vi "输入数据解析.vi"(0 "单个参数补充":dbl, 1 "从板号":dbl=1.0, 2 "主板二维码":string="BNET01", 3 "从板二维码":string="BNET01", 5 "主板引用":refnum<vi>, 7 "从板引用":refnum<vi>, 9 "主板选项":string="三级故障阀值", 11 "枚举":enum16{"主板", "从板"}(ring), 12 "快换":bool caption="快换写入") -> (4 "输出数组":dbl[][](array[numeric]), 6 "数组长度":dbl[](array[numeric]), 8 "循环次数":i32, 10 "命令":u32, 14 "名称":string[](array[string]), 15 "命令序号":u32[](array[numeric]))   [LabVIEW 2013]
panel:
  out "从板信息":T1
  out "主板数据":T2
  out "低位子数组 18":i32[](array[numeric])
  out "低位子数组 17":i32[](array[numeric])
  out "低位子数组 16":i32[](array[numeric])
  out "低位子数组 15":i32[](array[numeric])
  out "低位子数组 14":i32[](array[numeric])
  out "低位子数组 13":i32[](array[numeric])
  out "低位子数组 12":i32[](array[numeric])
  out "低位子数组 11":i32[](array[numeric])
  out "低位子数组 10":i32[](array[numeric])
  out "低位子数组 9":i32[](array[numeric])
  out "低位子数组 8":i32[](array[numeric])
  out "低位子数组 7":i32[](array[numeric])
  out "低位子数组 6":i32[](array[numeric])
  out "低位子数组 5":i32[](array[numeric])
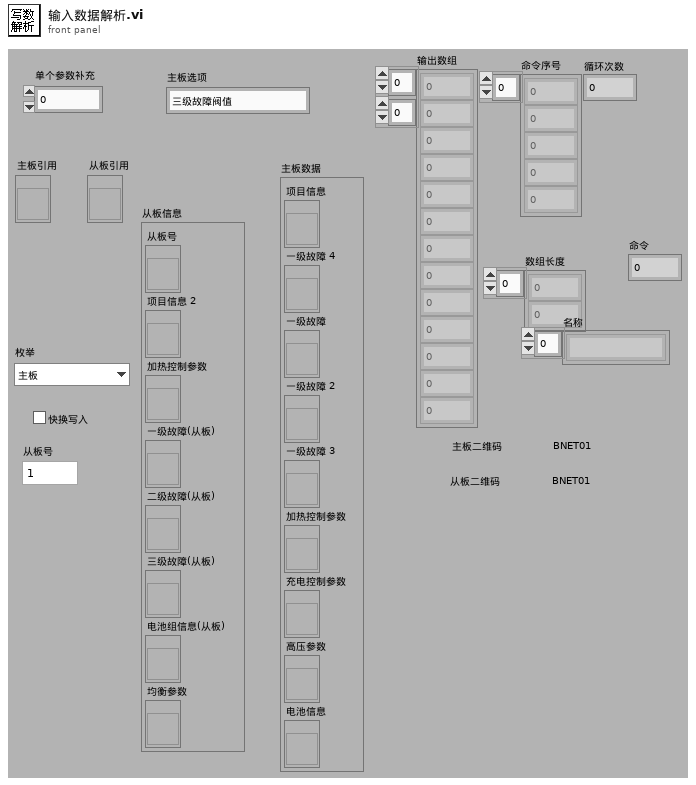
[diagram p1: front panel]
types:
  T1 = cluster{"从板号":refnum<vi>, "项目信息 2":refnum<vi>, "加热控制参数":refnum<vi>, "一级故障(从板)":refnum<vi>, "二级故障(从板)":refnum<vi>, "三级故障(从板)":refnum<vi>, "电池组信息(从板)":refnum<vi>, "均衡参数":refnum<vi>}
  T2 = cluster{"项目信息":refnum<vi>, "一级故障 4":refnum<vi>, "一级故障":refnum<vi>, "一级故障 2":refnum<vi>, "一级故障 3":refnum<vi>, "加热控制参数":refnum<vi>, "充电控制参数":refnum<vi>, "高压参数":refnum<vi>, "电池信息":refnum<vi>}
  T3 = cluster{"电池额定容量(A)":dbl, "使用者":dbl, "电池实际容量(A)":dbl, "车架(牌)号":string, "配置文件版本":string, "SOH(%)":dbl, "SOC(%)":dbl, "产品编号":string, "系统时钟":string}
  T4 = cluster{"总电压过高":dbl, "整组电压不均衡":dbl, "SOC过高":dbl, "单体电压过高":dbl, "总电压过低":dbl, "温度过高":dbl, "温度过低":dbl, "单组电压不均衡":dbl, "整组温度不均衡":dbl, "单组温度不均衡":dbl, "单体电压过低":dbl, "充电电流过高":dbl, "放电电流过高":dbl, "SOC过低":dbl, "内阻过大":dbl, "极柱温度过高":dbl, "SOH过低":dbl}
  T5 = cluster{"风机开启温度":dbl, "风机关闭温度":dbl, "加热开启温度":dbl, "加热关闭温度":dbl, "风机开启温差":dbl, "风机关闭温差":dbl, "加热关闭温差":dbl}
  T6 = cluster{"最大允许单体电压":dbl, "最大允许总电压":dbl, "最小允许单体电压":dbl, "最大允许充电电流":dbl, "最小允许充电电流":dbl, "最大允许充电温度":dbl, "最小允许充电温度":dbl, "电流步长":dbl}
  T7 = cluster{"电池串联":dbl, "电池并联":dbl, "累计放电总安时":dbl, "电池包额定容量":dbl, "电池包额定能量":dbl, "电池包额定总电压":dbl, "累计充电总安时":dbl, "电池充满次数":dbl, "电池放空次数":dbl, "电池充电次数":dbl, "电池生产日期":string, "电池厂家":string, "电池类型":string, "电池包组号":string, "电池包产权标识":string, "电池应用车型":string, "实际容量":dbl}
  T8 = cluster{"电压过高":dbl, "电压过低":dbl, "温度过高":dbl, "温度过低":dbl, "电压不均衡(V)":dbl, "温度不均衡":dbl, "SOC过低":dbl}
  T9 = cluster{"串联数":dbl, "并联数":dbl, "电池厂家":dbl, "电池类型":dbl, "额定能量":dbl, "额定容量":dbl, "实际容量":dbl, "额定总压":dbl, "产权标识":dbl, "应用车型":dbl, "电池包组号":dbl, "SOC":dbl, "充电总安时":dbl, "放电总这时":dbl, "放空次数":dbl, "充满次数":dbl, "充电次数":dbl, "车牌号":string, "生产日期":string, "最大允许单体电压":dbl, "最大允许总电压":dbl, "最大允许温度":dbl, "最小允许温度":dbl, "最大允许充电电流":dbl, "最小允许充电电流":dbl, "最小允许单体电压":dbl, "电流步长":dbl, "电池包序号":dbl}
  T10 = cluster{"充电结束电压(90%)":sgl, "充电结束电压(91%)":sgl, "充电结束电压(92%)":sgl, "充电结束电压(93%)":sgl, "充电结束电压(94%)":sgl, "均衡计算-电压高阀值1级":sgl, "均衡计算-电压高阀值2级":sgl, "均衡计算-电压低阀值1级":sgl, "均衡计算-电压低阀值2级":sgl, "均衡计算-最低电压阀值":sgl, "均衡停止-最低电压阀值":sgl, "均衡计算-电压极差阀值":sgl, "充电结束电压(95%)":sgl, "充电结束电压(96%)":sgl, "充电结束电压(97%)":sgl, "充电结束电压(98%)":sgl, "充电结束电压(99%)":sgl, "充电结束电压(100%)":sgl}
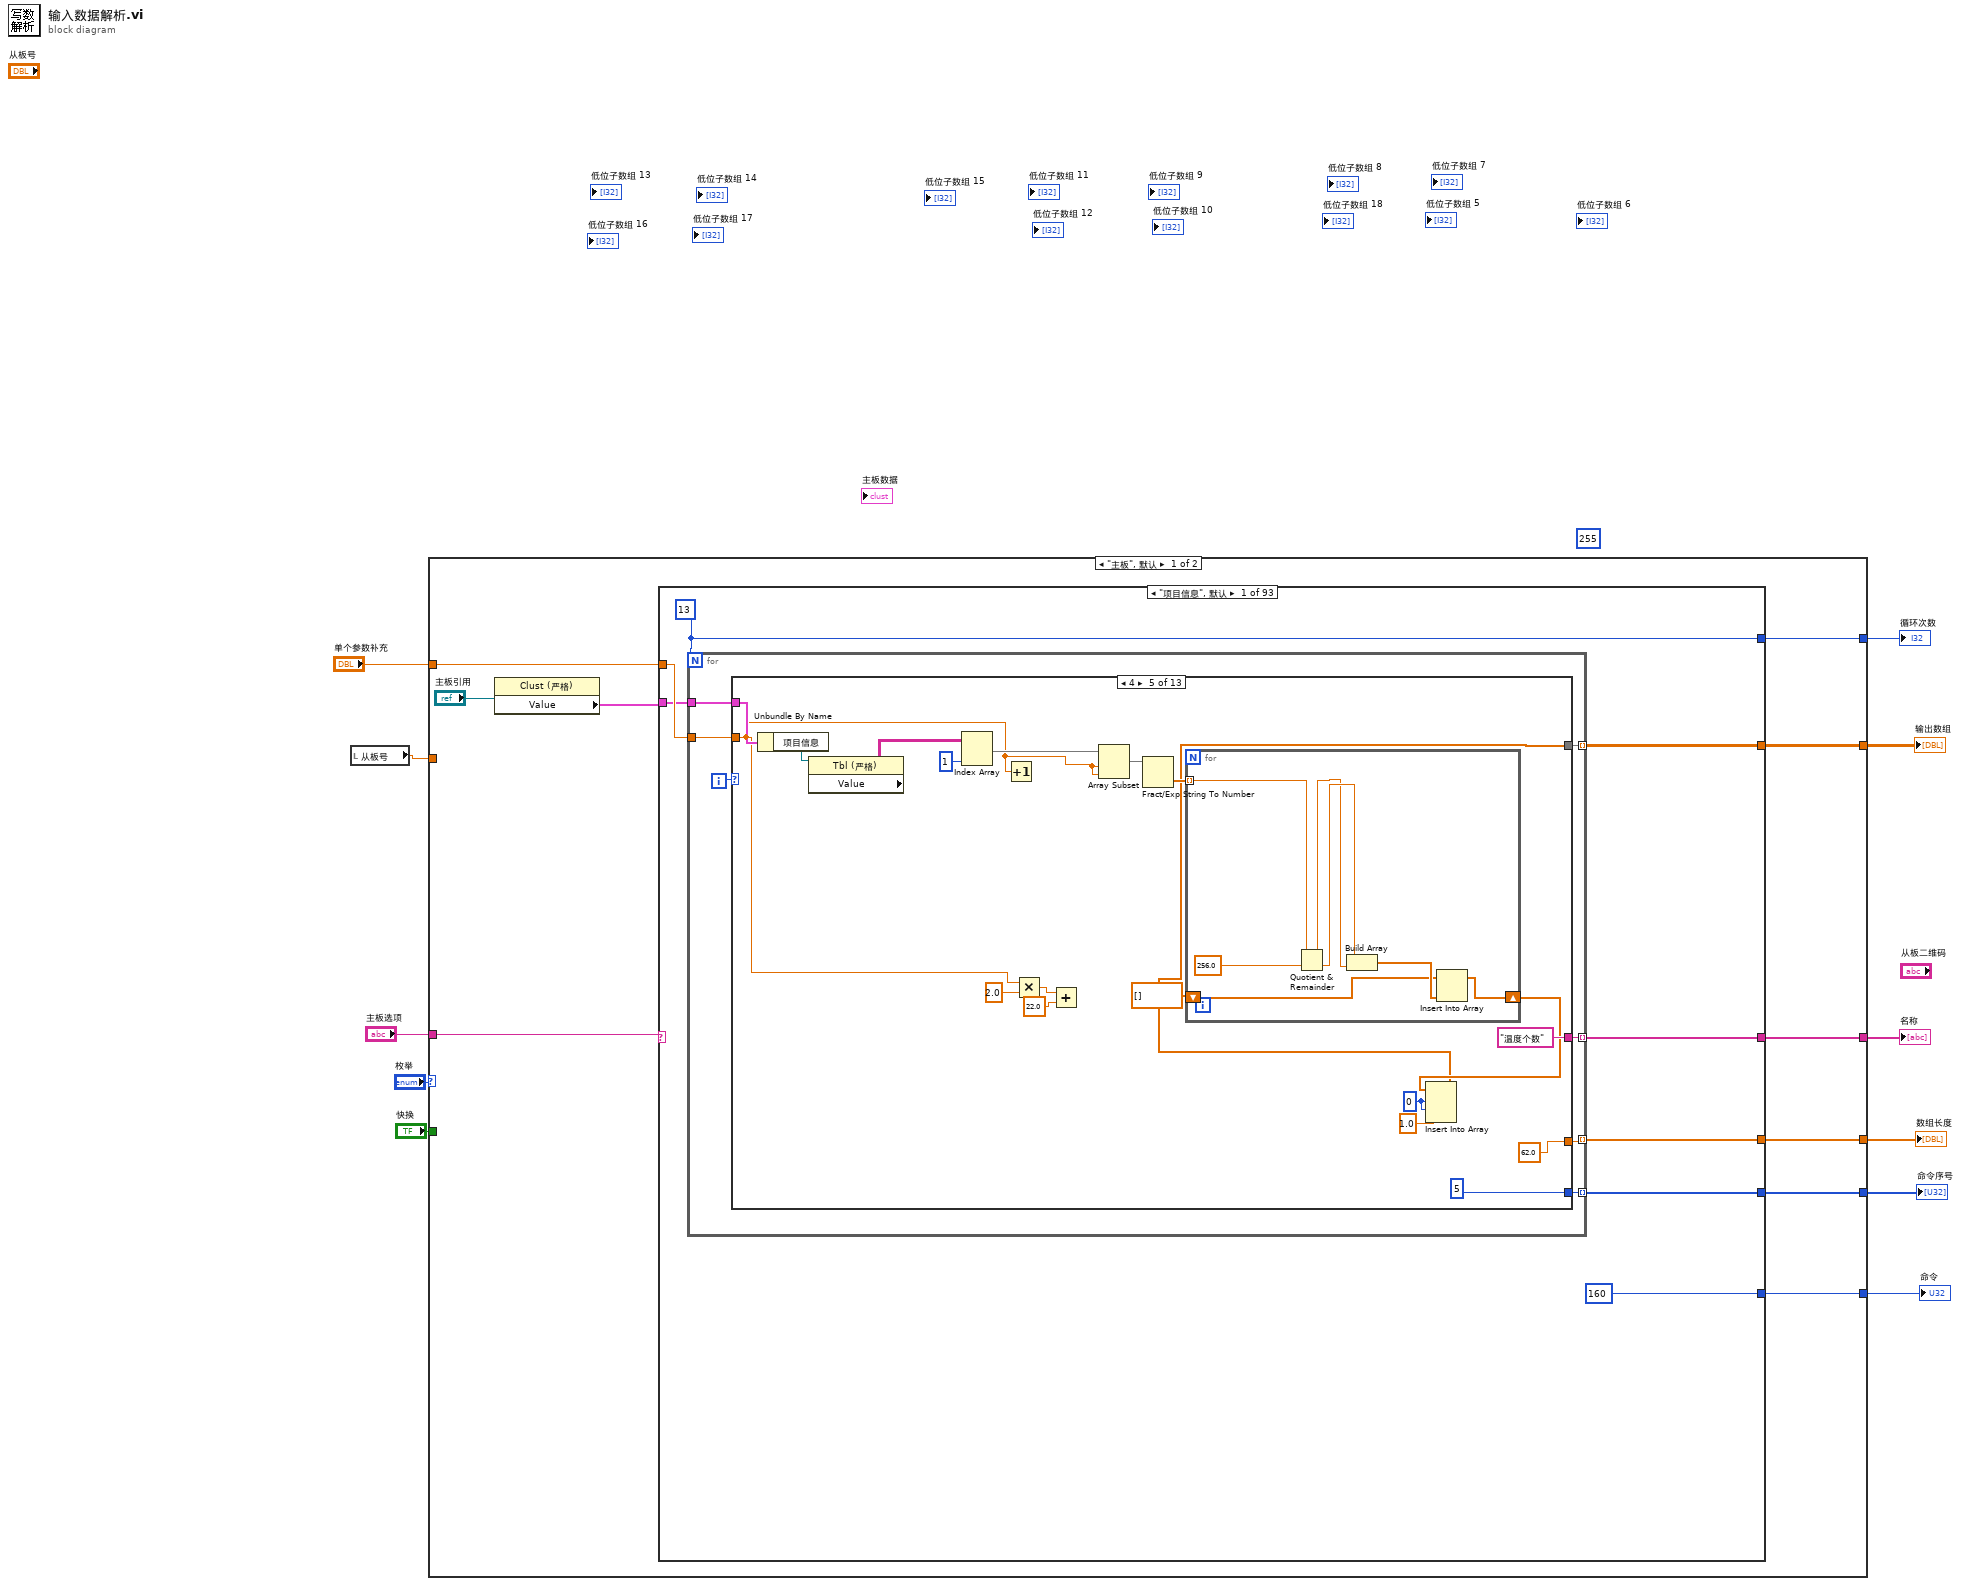
[diagram p0: block diagram]
diagram:
  (unwired) 255 ("高字节1")
  n1 = local read "从板号"() -> (w3:dbl)
  n2 = case shown="\"主板\", 默认" "枚举" {
    tunnel: "主板选项" -> [w21 w14872]
    tunnel: "单个参数补充" -> [w20 w14867]
    tunnel: [w19 w14871] -> w9
    tunnel: [w18 w14869] -> w8
    tunnel: [w17 w14868] -> w7
    tunnel: [w16 w14870] -> w6
    tunnel: "快换" -> [_ w14866]
    tunnel: w3 -> [_ w14865]
    tunnel: [w13 w14862] -> w2
    tunnel: [w12 w14861] -> w1
    frame "主板", Default {
      n3 = property class="Clust (严格)"(reference="主板引用") -> ("Value"=w14:T2)  [unwired: 1 in, 2 out]
      n4 = case shown="\"项目信息\", 默认" w21 {
        tunnel: w20 -> [w29 w289 _ _ w567 w599 w630 w651 w689 _ _ _ _ _ _ _ _ _ _ _ _ _ _ _ _ _ _ _ _ _ _ _ _ _ _ _ _ _ _ _ _ _ _ _ _ _ _ _ _ _ _ _ _ _ _ _ _ _ _ _ _ _ _ _ _ _ _ _ _ _ _ _ _ _ _ _ _ _ _ _ _ _ _ _ _ _ _ _ _ _ _ _ _]
        tunnel: w14 -> [w27 w287 w548 _ w586 w616 w643 w671 w702 w730 w767 w782 w806 _ w838 w856 w863 w1006 w1237 w1468 w1699 w1930 w2161 w2392 w2623 w2854 w3085 w3316 w3547 w3778 w4008 w4238 w4468 w4699 w4930 w5161 w5390 w5619 w5848 w6078 w6308 w6538 w6767 w6996 w7225 w7455 w7685 w7915 w8145 w8375 w8605 w8834 w9063 w9292 w9522 w9752 w9982 w10212 w10442 w10672 w10891 w11109 w11329 w11544 w11759 w11970 w12184 w12398 w12612 w12755 w12914 w12936 w12958 w12980 w13002 w13024 w13046 w13068 w13077 w13152 w13257 w13362 w13467 w13572 w13677 w13782 w13887 w13992 w14144 w14301 w14438 w14575 w14710]
        tunnel: [w28 w288 w535 w554 w571 w609 w636 w657 w683 w718 w738 w773 w789 w813 w829 w844 w867 w1010 w1241 w1472 w1703 w1934 w2165 w2396 w2627 w2858 w3089 w3320 w3551 w3782 w4012 w4242 w4472 w4703 w4934 w5165 w5394 w5623 w5852 w6082 w6312 w6542 w6771 w7000 w7229 w7459 w7689 w7919 w8149 w8379 w8609 w8838 w9067 w9296 w9526 w9756 w9986 w10216 w10446 w10676 w10895 w11113 w11333 w11548 w11763 w11974 w12188 w12402 w12616 w12759 w12918 w12940 w12962 w12984 w13006 w13028 w13050 w13072 w13084 w13159 w13264 w13369 w13474 w13579 w13684 w13789 w13894 w13994 w14146 w14303 w14440 w14577 w14709] -> w19
        tunnel: [w26 w286 w536 w555 w576 w606 w633 w662 w693 w716 w736 w771 w787 w811 w827 w842 u32[] [1] u32[] [1] u32[] [1] u32[] [1] u32[] [2] u32[] [3] u32[] [2] u32[] [3] u32[] [2] u32[] [3] u32[] [1] u32[] [2] u32[] [3] u32[] [1] u32[] [2] u32[] [3] u32[] [1] u32[] [2] u32[] [3] u32[] [1] u32[] [2] u32[] [3] u32[] [1] u32[] [2] u32[] [3] u32[] [1] u32[] [2] u32[] [3] u32[] [1] u32[] [2] u32[] [3] u32[] [1] u32[] [2] u32[] [3] u32[] [1] u32[] [2] u32[] [3] u32[] [1] u32[] [2] u32[] [3] u32[] [1] u32[] [2] u32[] [3] u32[] [1] u32[] [2] u32[] [3] u32[] [1] u32[] [2] u32[] [3] u32[] [1] u32[] [2] u32[] [3] u32[] [2] u32[] [3] u32[] [1] u32[] [1] u32[] [1] u32[] [1] u32[] [1] u32[] [1] u32[] [1] u32[] [1] u32[] [2] u32[] [2] u32[] [2] u32[] [2] u32[] [2] u32[] [2] u32[] [2] u32[] [2] u32[] [2] w13996 w14148 w14305 w14442 w14579 w14711] -> w18
        tunnel: [w25 w285 w537 w556 w578 w608 w635 w664 w695 w717 w737 w772 w788 w812 w828 w843 dbl[] [28.0] dbl[] [28.0] dbl[] [28.0] dbl[] [28.0] dbl[] [28.0] dbl[] [28.0] dbl[] [28.0] dbl[] [28.0] dbl[] [28.0] dbl[] [28.0] dbl[] [28.0] dbl[] [28.0] dbl[] [28.0] dbl[] [28.0] dbl[] [28.0] dbl[] [28.0] dbl[] [28.0] dbl[] [28.0] dbl[] [28.0] dbl[] [28.0] dbl[] [28.0] dbl[] [28.0] dbl[] [28.0] dbl[] [28.0] dbl[] [28.0] dbl[] [28.0] dbl[] [28.0] dbl[] [28.0] dbl[] [28.0] dbl[] [28.0] dbl[] [28.0] dbl[] [28.0] dbl[] [28.0] dbl[] [28.0] dbl[] [28.0] dbl[] [28.0] dbl[] [28.0] dbl[] [28.0] dbl[] [28.0] dbl[] [28.0] dbl[] [28.0] dbl[] [28.0] dbl[] [28.0] dbl[] [28.0] dbl[] [28.0] dbl[] [28.0] dbl[] [28.0] dbl[] [28.0] dbl[] [28.0] dbl[] [28.0] dbl[] [28.0] dbl[] [28.0] dbl[] [28.0] dbl[] [28.0] dbl[] [7.0] dbl[] [7.0] dbl[] [7.0] dbl[] [7.0] dbl[] [7.0] dbl[] [7.0] dbl[] [7.0] dbl[] [7.0] dbl[] [14.0] dbl[] [14.0] dbl[] [14.0] dbl[] [14.0] dbl[] [14.0] dbl[] [14.0] dbl[] [14.0] dbl[] [14.0] dbl[] [14.0] w13997 w14149 w14306 w14443 w14580 w14712] -> w17
        tunnel: [u32 160 ("命令序号") u32 160 ("命令序号") u32 160 ("命令序号") u32 172 ("命令序号") u32 160 ("命令序号") u32 160 ("命令序号") u32 160 ("命令序号") u32 160 ("命令序号") u32 160 ("命令序号") u32 160 ("命令序号") u32 160 ("命令序号") u32 160 ("命令序号") u32 160 ("命令序号") u32 160 ("命令序号") u32 160 ("命令序号") u32 160 ("命令序号") u32 161 ("命令序号") u32 161 ("命令序号") u32 161 ("命令序号") u32 161 ("命令序号") u32 161 ("命令序号") u32 161 ("命令序号") u32 161 ("命令序号") u32 161 ("命令序号") u32 161 ("命令序号") u32 161 ("命令序号") u32 161 ("命令序号") u32 161 ("命令序号") u32 161 ("命令序号") u32 161 ("命令序号") u32 161 ("命令序号") u32 161 ("命令序号") u32 161 ("命令序号") u32 161 ("命令序号") u32 161 ("命令序号") u32 161 ("命令序号") u32 161 ("命令序号") u32 161 ("命令序号") u32 161 ("命令序号") u32 161 ("命令序号") u32 161 ("命令序号") u32 161 ("命令序号") u32 161 ("命令序号") u32 161 ("命令序号") u32 161 ("命令序号") u32 161 ("命令序号") u32 161 ("命令序号") u32 161 ("命令序号") u32 161 ("命令序号") u32 161 ("命令序号") u32 161 ("命令序号") u32 161 ("命令序号") u32 161 ("命令序号") u32 161 ("命令序号") u32 161 ("命令序号") u32 161 ("命令序号") u32 161 ("命令序号") u32 161 ("命令序号") u32 161 ("命令序号") u32 161 ("命令序号") u32 161 ("命令序号") u32 161 ("命令序号") u32 161 ("命令序号") u32 161 ("命令序号") u32 161 ("命令序号") u32 161 ("命令序号") u32 161 ("命令序号") u32 161 ("命令序号") u32 161 ("命令序号") u32 161 ("命令序号") u32 162 ("命令序号") u32 162 ("命令序号") u32 162 ("命令序号") u32 162 ("命令序号") u32 162 ("命令序号") u32 162 ("命令序号") u32 162 ("命令序号") u32 162 ("命令序号") u32 162 ("命令序号") u32 162 ("命令序号") u32 162 ("命令序号") u32 162 ("命令序号") u32 162 ("命令序号") u32 162 ("命令序号") u32 162 ("命令序号") u32 162 ("命令序号") u32 162 ("命令序号") u32 164 ("命令序号") u32 164 ("命令序号") u32 164 ("命令序号") u32 164 ("命令序号") u32 164 ("命令序号") w14713] -> w16
        tunnel: [w23 w283 1 1 1 1 1 1 1 w726 1 1 1 1 1 1 1 1 1 1 1 1 1 1 1 1 1 1 1 1 1 1 1 1 1 1 1 1 1 1 1 1 1 1 1 1 1 1 1 1 1 1 1 1 1 1 1 1 1 1 1 1 1 1 1 1 1 1 1 1 1 1 1 1 1 1 1 1 1 1 1 1 1 1 1 1 1 1 4 1 1 1 _] -> w13
        tunnel: [w22 w282 w542 w558 w568 w595 w626 w653 w679 w714 w734 w769 w784 w808 w825 w840 w858 w1001 w1232 w1463 w1694 w1925 w2156 w2387 w2618 w2849 w3080 w3311 w3542 w3773 w4003 w4233 w4463 w4694 w4925 w5156 w5385 w5614 w5843 w6073 w6303 w6533 w6762 w6991 w7220 w7450 w7680 w7910 w8140 w8370 w8600 w8829 w9058 w9287 w9517 w9747 w9977 w10207 w10437 w10667 w10886 w11104 w11324 w11539 w11754 w11965 w12179 w12393 w12607 w12750 string[] ["加热控制参数"] string[] ["加热控制参数"] string[] ["加热控制参数"] string[] ["加热控制参数"] string[] ["加热控制参数"] string[] ["加热控制参数"] string[] ["加热控制参数"] string[] ["加热控制参数"] string[] ["充电控制参数"] string[] ["充电控制参数"] string[] ["充电控制参数"] string[] ["充电控制参数"] string[] ["充电控制参数"] string[] ["充电控制参数"] string[] ["充电控制参数"] string[] ["充电控制参数"] string[] ["充电控制参数"] string[] ["电池信息1"] w14141 string[] ["电池包组号"] string[] ["充放电安时"] string[] ["电池充放电次数"] _] -> w12
        frame "项目信息", Default {
          w23 = 13
          n5 = for {
            N: w23 -> [_]
            tunnel: w29 -> [w36]
            tunnel: [w35] -> w28 mode=indexing
            tunnel: [w34] -> w26 mode=indexing
            tunnel: w27 -> [w33]
            tunnel: [w32] -> w25 mode=indexing
            tunnel: [w31] -> w22 mode=indexing
            i -> [w30]
            n6 = case shown="4" w30 {
              tunnel: w36 -> [_ w48 w77 w92 w116 w142 w170 _ _ _ _ _ _]
              tunnel: [w43 w51 w71 w91 w114 w140 w163 w221 w233 w240 w246 w267 w281] -> w35
              tunnel: [u32 1 ("命令序号") u32 2 ("命令序号") u32 3 ("命令序号") u32 4 ("命令序号") u32 5 ("命令序号") u32 6 ("命令序号") u32 13 ("命令序号") u32 8 ("命令序号") u32 7 ("命令序号") u32 9 ("命令序号") u32 10 ("命令序号") u32 11 ("命令序号") u32 12 ("命令序号")] -> w34
              tunnel: w33 -> [w41 w52 w76 w93 w117 w141 w169 w202 w229 w237 w247 w264 w277]
              tunnel: [w42 63.0 ("单个参数补充") 20.0 ("单个参数补充") 62.0 ("元素") 62.0 ("元素") 62.0 ("元素") 10.0 ("元素") 8.0 ("单个参数补充") 2.0 ("单个参数补充") w239 8.0 ("单个参数补充") w266 2.0 ("单个参数补充")] -> w32
              tunnel: ["产品编号" "电压个数" "通道电压数" "电压起始值" "温度个数" "温度起始值" "保险位置" "电池额定实际容量" "SOC" "配置文件版本" "参数修改记录" "车牌号" "SOH"] -> w31
              frame 0, Default {
                w42 = 16 ("长度")
                # "产品编号"
                n7 = Unbundle By Name(w41) -> ("一级故障 4"=w40:refnum<vi>)
                n8 = property class="Clust (严格)"(reference=w40) -> ("Value"=w39:T3)  [unwired: 1 in, 2 out]
                n9 = Unbundle By Name(w39) -> ("产品编号"=w38:string)
                n10 = String To Byte Array(string=w38) -> (unsigned byte array=w44:u8[])
                n11 = Array Subset(array=w44, length=w42) -> (w43:u8[])  [unwired: 1 in]
              }
              frame 1 {
                # "电压个数"
                # "电压个数"
                n12 = Unbundle By Name(w52) -> ("项目信息"=w57:refnum<vi>)
                n13 = property class="Tbl (严格)"(reference=w57) -> ("Value"=w56:string[][])  [unwired: 1 in, 2 out]
                n14 = Index Array(array=w56, index (col)=1 ("禁用的索引 (列)")) -> (element=w58:string[])  [unwired: 1 in]
                n15 = Array Subset(array=w58, index=0 ("索引"), length=w48) -> (w61:string[])
                n16 = Fract/Exp String To Number(string=w61) -> (number=w55:dbl[])  [unwired: 4 out]
                n17 = for {
                  tunnel: w55 -> [w70] mode=indexing
                  shift-right: [w65] -> w53
                  shift-left: dbl[] [] -> [w64]
                  n18 = Quotient & Remainder(x=w70, y=256.0) -> (x-y*floor(x/y)=w67:dbl, floor(x/y)=w68:dbl)
                  n19 = Build Array(w68, w67) -> (w66:dbl[])
                  n20 = Insert Into Array(array=w64, new element=w66) -> (w65:dbl[])  [unwired: 1 in]
                }
                n21 = Insert Into Array(array=w53, index=0 ("索引"), new element #1=w48, new element #2=0.0 ("新元素/子数组"), new element #3=1.0 ("新元素/子数组")) -> (w51:dbl[])
              }
              frame 2 {
                # "全部给1"
                n22 = Unbundle By Name(w76) -> ("项目信息"=w81:refnum<vi>)
                n23 = property class="Tbl (严格)"(reference=w81) -> ("Value"=w80:string[][])  [unwired: 1 in, 2 out]
                n24 = Index Array(array=w80, index (col)=1 ("禁用的索引 (列)")) -> (element=w82:string[])  [unwired: 1 in]
                n25 = Increment(x=w77) -> (x+1=w78:dbl)
                n26 = Array Subset(array=w82, index=w78, length=20 ("长度")) -> (w84:string[])
                n27 = Fract/Exp String To Number(string=w84) -> (number=w72:dbl[])  [unwired: 4 out]
                n28 = for {
                  tunnel: [1.0 ("y")] -> w71 mode=indexing
                  tunnel: w72 -> [w86] mode=indexing
                  w87 = 12.0 ("y")
                  n29 = Greater?(x=w86, y=w87) -> (0:w88:bool)
                  n30 = Select(t=w87, s=w88, f=w86) -> ()  [unwired: 1 out]
                }
              }
              frame 3 {
                # "全部给1"
                # "电压起始值"
                n31 = Unbundle By Name(w93) -> ("项目信息"=w100:refnum<vi>)
                n32 = property class="Tbl (严格)"(reference=w100) -> ("Value"=w99:string[][])  [unwired: 1 in, 2 out]
                n33 = Index Array(array=w99, index (col)=1 ("禁用的索引 (列)")) -> (element=w101:string[])  [unwired: 1 in]
                n34 = Add(x=21.0, y=w92) -> (x+y=w96:dbl)
                n35 = Increment(x=w92) -> (x+1=w94:dbl)
                n36 = Array Subset(array=w101, index=w96, length=w94) -> (w103:string[])
                n37 = Fract/Exp String To Number(string=w103) -> (number=w98:dbl[])  [unwired: 4 out]
                n38 = for {
                  tunnel: w98 -> [w111] mode=indexing
                  shift-right: [w108] -> w91
                  shift-left: dbl[] [] -> [w107]
                  n39 = Quotient & Remainder(x=w111, y=256.0) -> ()  [unwired: 2 out]
                  n40 = Build Array(0.0 ("元素"), 1.0 ("元素")) -> (w109:dbl[])
                  n41 = Insert Into Array(array=w107, new element=w109) -> (w108:dbl[])  [unwired: 1 in]
                }
              }
              frame 4 {
                w113 = 0 ("索引")
                n42 = Unbundle By Name(w117) -> ("项目信息"=w124:refnum<vi>)
                n43 = property class="Tbl (严格)"(reference=w124) -> ("Value"=w123:string[][])  [unwired: 1 in, 2 out]
                n44 = Index Array(array=w123, index (col)=1 ("禁用的索引 (列)")) -> (element=w125:string[])  [unwired: 1 in]
                n45 = Increment(x=w116) -> ()  [unwired: 1 out]
                n46 = Multiply(x=w116, y=2.0) -> (x*y=w121:dbl)
                n47 = Add(x=w121, y=22.0) -> ()  [unwired: 1 out]
                n48 = Array Subset(array=w125, index=w116, length=w116) -> (w127:string[])
                n49 = Fract/Exp String To Number(string=w127) -> (number=w119:dbl[])  [unwired: 4 out]
                n50 = for {
                  tunnel: w119 -> [w137] mode=indexing
                  shift-right: [w132] -> w115
                  shift-left: dbl[] [] -> [w131]
                  n51 = Quotient & Remainder(x=w137, y=256.0) -> (x-y*floor(x/y)=w134:dbl, floor(x/y)=w135:dbl)
                  n52 = Build Array(w135, w134) -> (w133:dbl[])
                  n53 = Insert Into Array(array=w131, new element=w133) -> (w132:dbl[])  [unwired: 1 in]
                }
                n54 = Insert Into Array(array=w115, index=w113, new element #1=w113, new element #2=1.0 ("新元素/子数组")) -> (w114:dbl[])
              }
              frame 5 {
                # "全部给1"
                n55 = Unbundle By Name(w141) -> ("项目信息"=w151:refnum<vi>)
                n56 = property class="Tbl (严格)"(reference=w151) -> ("Value"=w150:string[][])  [unwired: 1 in, 2 out]
                n57 = Index Array(array=w150, index (col)=1 ("禁用的索引 (列)")) -> (element=w152:string[])  [unwired: 1 in]
                n58 = Increment(x=w142) -> (x+1=w149:dbl)
                n59 = Multiply(x=w142, y=3.0) -> (x*y=w146:dbl)
                n60 = Add(x=w146, y=23.0) -> (x+y=w148:dbl)
                n61 = Array Subset(array=w152, index=w148, length=w149) -> (w154:string[])
                n62 = Fract/Exp String To Number(string=w154) -> (number=w144:dbl[])  [unwired: 4 out]
                n63 = for {
                  tunnel: w144 -> [w162] mode=indexing
                  shift-right: [w159] -> w140
                  shift-left: dbl[] [] -> [w158]
                  n64 = Quotient & Remainder(x=w162, y=256.0) -> ()  [unwired: 2 out]
                  n65 = Build Array(0.0 ("元素"), 1.0 ("元素")) -> (w160:dbl[])
                  n66 = Insert Into Array(array=w158, new element=w160) -> (w159:dbl[])  [unwired: 1 in]
                }
              }
              frame 6 {
                n67 = Unbundle By Name(w169) -> ("项目信息"=w176:refnum<vi>)
                n68 = property class="Tbl (严格)"(reference=w176) -> ("Value"=w175:string[][])  [unwired: 1 in, 2 out]
                n69 = Multiply(x=w170, y=4.0) -> (x*y=w172:dbl)
                n70 = Add(x=w172, y=24.0) -> (x+y=w174:dbl)
                n71 = Index Array(array=w175, index (col)=1 ("禁用的索引 (列)")) -> (element=w177:string[])  [unwired: 1 in]
                n72 = Array Subset(array=w177, index=w174, length=20 ("长度")) -> (w179:string[])
                n73 = Fract/Exp String To Number(string=w179) -> (number=w165:dbl[])  [unwired: 4 out]
                n74 = for {
                  N: 10 -> [_]
                  tunnel: w165 -> [w190]
                  tunnel: [0] -> w163 mode=indexing
                  i -> [w192]
                  w185 = 4 ("索引")
                  n75 = Multiply(x=w192, y=2) -> (x*y=w189:i32)
                  n76 = Increment(x=w189) -> (x+1=w188:i32)
                  n77 = Index Array(array=w190, index #1=w189, index #2=w188) -> (element #1=w187:dbl, element #2=w186:dbl)
                  n78 = call "二进制解析-8.6.vi"("索引"=w185, "数值"=w187) -> ("低位子数组"=w184:i32[])  [unwired: 1 in, 2 out]
                  n79 = call "二进制解析-8.6.vi"("索引"=w185, "数值"=w186) -> ("低位子数组"=w183:i32[])  [unwired: 1 in, 2 out]
                  n80 = Insert Into Array(array=w184, new element=w183) -> (w182:i32[])  [unwired: 1 in]
                  n81 = call "数值二进制转十进制-8.6.vi"("子数组"=w182) -> ()  [unwired: 4 in, 1 out]
                }
              }
              frame 7 {
                w211 = 256.0 ("y")
                w213 = 256.0 ("y")
                # "电池额定容量,实际容量"
                n82 = Unbundle By Name(w202) -> ("一级故障 4"=w201:refnum<vi>)
                n83 = property class="Clust (严格)"(reference=w201) -> ("Value"=w200:T3)  [unwired: 1 in, 2 out]
                n84 = Unbundle By Name(w200) -> ("电池额定容量(A)"=w198:dbl, "电池实际容量(A)"=w197:dbl)
                n85 = call "输入分辨率计算-EV05.vi"("1字节?"=TRUE, "数值 2"=w197, "数值"=w198, "分辨率"=0.001) -> ("高字节 2"=w195:dbl, "高字节1"=w196:dbl)  [unwired: 1 in, 5 out]
                n86 = Quotient & Remainder(x=w196, y=w213) -> (x-y*floor(x/y)=w217:dbl, floor(x/y)=w219:dbl)
                n87 = Quotient & Remainder(x=w195, y=w211) -> (x-y*floor(x/y)=w204:dbl, floor(x/y)=w208:dbl)
                n88 = Quotient & Remainder(x=w219, y=w213) -> (x-y*floor(x/y)=w216:dbl, floor(x/y)=w218:dbl)
                n89 = Quotient & Remainder(x=w208, y=w211) -> (x-y*floor(x/y)=w205:dbl, floor(x/y)=w209:dbl)
                n90 = Quotient & Remainder(x=w218, y=w213) -> (x-y*floor(x/y)=w215:dbl, floor(x/y)=w214:dbl)
                n91 = Quotient & Remainder(x=w209, y=w211) -> (x-y*floor(x/y)=w206:dbl, floor(x/y)=w210:dbl)
                n92 = Quotient & Remainder(x=w214, y=w213) -> (x-y*floor(x/y)=w212:dbl)  [unwired: 1 out]
                n93 = Quotient & Remainder(x=w210, y=w211) -> (x-y*floor(x/y)=w207:dbl)  [unwired: 1 out]
                n94 = Build Array(w212, w215, w216, w217, w207, w206, w205, w204) -> (w221:dbl[])
              }
              frame 8 {
                # "SOC"
                n95 = Unbundle By Name(w229) -> ("一级故障 4"=w230:refnum<vi>)
                n96 = property class="Clust (严格)"(reference=w230) -> ("Value"=w228:T3)  [unwired: 1 in, 2 out]
                n97 = Unbundle By Name(w228) -> ("SOC(%)"=w226:dbl)
                n98 = call "输入分辨率计算-EV05.vi"("1字节?"=FALSE, "数值"=w226, "分辨率"=0.1) -> ("低字节"=w223:dbl, "高字节1"=w224:dbl)  [unwired: 2 in, 5 out]
                n99 = Build Array(w224, w223) -> (w233:dbl[])
              }
              frame 9 {
                w239 = 8 ("长度")
                # "配置文件版本"
                n100 = Unbundle By Name(w237) -> ("一级故障 4"=w238:refnum<vi>)
                n101 = property class="Clust (严格)"(reference=w238) -> ("Value"=w236:T3)  [unwired: 1 in, 2 out]
                n102 = Unbundle By Name(w236) -> ("配置文件版本"=w235:string)
                n103 = String To Byte Array(string=w235) -> (unsigned byte array=w241:u8[])
                n104 = Array Subset(array=w241, length=w239) -> (w240:u8[])  [unwired: 1 in]
              }
              frame 10 {
                n105 = Unbundle By Name(w247) -> ("一级故障 4"=w253:refnum<vi>)
                n106 = property class="Clust (严格)"(reference=w253) -> ("Value"=w252:T3)  [unwired: 1 in, 2 out]
                n107 = Unbundle By Name(w252) -> ("使用者"=w251:dbl)
                n108 = Quotient & Remainder(x=w251, y=256.0) -> (x-y*floor(x/y)=w248:dbl, floor(x/y)=w249:dbl)
                n109 = call "当前时间解析-8.6.vi"("需要秒？(T)"=TRUE) -> ("年"=w259:u8, "月"=w258:u8, "日"=w257:u8, "时"=w256:u8, "分"=w255:u8, "秒"=w254:u8)  [unwired: 13 out]
                n110 = Build Array(w249, w248, w259, w258, w257, w256, w255, w254) -> (w246:dbl[])
              }
              frame 11 {
                w266 = 8 ("长度")
                # "车牌号"
                n111 = Unbundle By Name(w264) -> ("一级故障 4"=w265:refnum<vi>)
                n112 = property class="Clust (严格)"(reference=w265) -> ("Value"=w263:T3)  [unwired: 1 in, 2 out]
                n113 = Unbundle By Name(w263) -> ("车架(牌)号"=w262:string)
                n114 = String To Byte Array(string=w262) -> (unsigned byte array=w268:u8[])
                n115 = Array Subset(array=w268, length=w266) -> (w267:u8[])  [unwired: 1 in]
              }
              frame 12 {
                # "SOH"
                n116 = Unbundle By Name(w277) -> ("一级故障 4"=w278:refnum<vi>)
                n117 = property class="Clust (严格)"(reference=w278) -> ("Value"=w276:T3)  [unwired: 1 in, 2 out]
                n118 = Unbundle By Name(w276) -> ("SOH(%)"=w275:dbl)
                n119 = call "输入分辨率计算-EV05.vi"("1字节?"=FALSE, "数值"=w275, "分辨率"=0.1) -> ("低字节"=w271:dbl, "高字节1"=w272:dbl)  [unwired: 2 in, 5 out]
                n120 = Build Array(w272, w271) -> (w281:dbl[])
              }
            }
          }
        }
        frame "保险位置" {
          w283 = 1
          n121 = for {
            N: w283 -> [_]
            tunnel: w289 -> [w296]
            tunnel: [w295] -> w288 mode=indexing
            tunnel: [w294] -> w286 mode=indexing
            tunnel: w287 -> [w293]
            tunnel: [w292] -> w285 mode=indexing
            tunnel: [w291] -> w282 mode=indexing
            i -> [w290]
            n122 = case shown="9" w290 {
              tunnel: w296 -> [w304 w330 w356 w367 w389 w416 _ _ _ _ _ _ _]
              tunnel: [w298 w329 w355 w366 w387 w414 w443 w474 w486 w493 w499 w520 w534] -> w295
              tunnel: [u32 13 ("命令序号") u32 2 ("命令序号") u32 3 ("命令序号") u32 4 ("命令序号") u32 5 ("命令序号") u32 6 ("命令序号") u32 1 ("命令序号") u32 8 ("命令序号") u32 7 ("命令序号") u32 9 ("命令序号") u32 10 ("命令序号") u32 11 ("命令序号") u32 12 ("命令序号")] -> w294
              tunnel: w293 -> [w303 w331 w354 w368 w388 w415 w441 w455 w482 w490 w500 w517 w530]
              tunnel: [10.0 ("元素") 63.0 ("单个参数补充") 20.0 ("单个参数补充") 62.0 ("元素") 62.0 ("元素") 62.0 ("元素") w442 8.0 ("单个参数补充") 2.0 ("单个参数补充") w492 8.0 ("单个参数补充") w519 2.0 ("单个参数补充")] -> w292
              tunnel: ["保险位置" "电压个数" "通道电压数" "电压起始值" "温度个数" "温度起始值" "产品编号" "电池额定实际容量" "SOC" "配置文件版本" "参数修改记录" "车牌号" "SOH"] -> w291
              frame 0, Default {
                n123 = Unbundle By Name(w303) -> ("项目信息"=w310:refnum<vi>)
                n124 = property class="Tbl (严格)"(reference=w310) -> ("Value"=w309:string[][])  [unwired: 1 in, 2 out]
                n125 = Multiply(x=w304, y=4.0) -> (x*y=w306:dbl)
                n126 = Add(x=w306, y=24.0) -> (x+y=w308:dbl)
                n127 = Index Array(array=w309, index (col)=1 ("禁用的索引 (列)")) -> (element=w311:string[])  [unwired: 1 in]
                n128 = Array Subset(array=w311, index=w308, length=20 ("长度")) -> (w313:string[])
                n129 = Fract/Exp String To Number(string=w313) -> (number=w299:dbl[])  [unwired: 4 out]
                n130 = for {
                  N: 10 -> [_]
                  tunnel: w299 -> [w324]
                  tunnel: [w315] -> w298 mode=indexing
                  i -> [w326]
                  w319 = 4 ("索引")
                  n131 = Multiply(x=w326, y=2) -> (x*y=w323:i32)
                  n132 = Increment(x=w323) -> (x+1=w322:i32)
                  n133 = Index Array(array=w324, index #1=w323, index #2=w322) -> (element #1=w321:dbl, element #2=w320:dbl)
                  n134 = call "二进制解析-8.6.vi"("索引"=w319, "数值"=w321) -> ("低位子数组"=w318:i32[])  [unwired: 1 in, 2 out]
                  n135 = call "二进制解析-8.6.vi"("索引"=w319, "数值"=w320) -> ("低位子数组"=w317:i32[])  [unwired: 1 in, 2 out]
                  n136 = Insert Into Array(array=w318, new element=w317) -> (w316:i32[])  [unwired: 1 in]
                  n137 = call "数值二进制转十进制-8.6.vi"("子数组"=w316) -> ("十进制数值"=w315:i32)  [unwired: 4 in]
                }
              }
              frame 1 {
                # "电压个数"
                # "电压个数"
                n138 = Unbundle By Name(w331) -> ("项目信息"=w337:refnum<vi>)
                n139 = property class="Tbl (严格)"(reference=w337) -> ("Value"=w336:string[][])  [unwired: 1 in, 2 out]
                n140 = Index Array(array=w336, index (col)=1 ("禁用的索引 (列)")) -> (element=w338:string[])  [unwired: 1 in]
                n141 = Increment(x=w330) -> (x+1=w332:dbl)
                n142 = Array Subset(array=w338, index=0 ("索引"), length=w332) -> (w341:string[])
                n143 = Fract/Exp String To Number(string=w341) -> (number=w335:dbl[])  [unwired: 4 out]
                n144 = for {
                  tunnel: w335 -> [w350] mode=indexing
                  shift-right: [w345] -> w333
                  shift-left: dbl[] [] -> [w344]
                  n145 = Quotient & Remainder(x=w350, y=256.0) -> (x-y*floor(x/y)=w347:dbl, floor(x/y)=w348:dbl)
                  n146 = Build Array(w348, w347) -> (w346:dbl[])
                  n147 = Insert Into Array(array=w344, new element=w346) -> (w345:dbl[])  [unwired: 1 in]
                }
                n148 = Insert Into Array(array=w333, index=0 ("索引"), new element=w330) -> (w329:dbl[])
              }
              frame 2 {
                n149 = Unbundle By Name(w354) -> ("项目信息"=w360:refnum<vi>)
                n150 = property class="Tbl (严格)"(reference=w360) -> ("Value"=w359:string[][])  [unwired: 1 in, 2 out]
                n151 = Index Array(array=w359, index (col)=1 ("禁用的索引 (列)")) -> (element=w361:string[])  [unwired: 1 in]
                n152 = Increment(x=w356) -> (x+1=w357:dbl)
                n153 = Array Subset(array=w361, index=w357, length=20 ("长度")) -> (w363:string[])
                n154 = Fract/Exp String To Number(string=w363) -> (number=w355:dbl[])  [unwired: 4 out]
              }
              frame 3 {
                # "电压起始值"
                n155 = Unbundle By Name(w368) -> ("项目信息"=w375:refnum<vi>)
                n156 = property class="Tbl (严格)"(reference=w375) -> ("Value"=w374:string[][])  [unwired: 1 in, 2 out]
                n157 = Index Array(array=w374, index (col)=1 ("禁用的索引 (列)")) -> (element=w376:string[])  [unwired: 1 in]
                n158 = Add(x=21.0, y=w367) -> (x+y=w371:dbl)
                n159 = Increment(x=w367) -> (x+1=w369:dbl)
                n160 = Array Subset(array=w376, index=w371, length=w369) -> (w378:string[])
                n161 = Fract/Exp String To Number(string=w378) -> (number=w373:dbl[])  [unwired: 4 out]
                n162 = for {
                  tunnel: w373 -> [w386] mode=indexing
                  shift-right: [w381] -> w366
                  shift-left: dbl[] [] -> [w380]
                  n163 = Quotient & Remainder(x=w386, y=256.0) -> (x-y*floor(x/y)=w383:dbl, floor(x/y)=w384:dbl)
                  n164 = Build Array(w384, w383) -> (w382:dbl[])
                  n165 = Insert Into Array(array=w380, new element=w382) -> (w381:dbl[])  [unwired: 1 in]
                }
              }
              frame 4 {
                n166 = Unbundle By Name(w388) -> ("项目信息"=w398:refnum<vi>)
                n167 = property class="Tbl (严格)"(reference=w398) -> ("Value"=w397:string[][])  [unwired: 1 in, 2 out]
                n168 = Index Array(array=w397, index (col)=1 ("禁用的索引 (列)")) -> (element=w399:string[])  [unwired: 1 in]
                n169 = Increment(x=w389) -> (x+1=w396:dbl)
                n170 = Multiply(x=w389, y=2.0) -> (x*y=w393:dbl)
                n171 = Add(x=w393, y=22.0) -> (x+y=w395:dbl)
                n172 = Array Subset(array=w399, index=w395, length=w396) -> (w401:string[])
                n173 = Fract/Exp String To Number(string=w401) -> (number=w391:dbl[])  [unwired: 4 out]
                n174 = for {
                  tunnel: w391 -> [w411] mode=indexing
                  shift-right: [w406] -> w387
                  shift-left: dbl[] [] -> [w405]
                  n175 = Quotient & Remainder(x=w411, y=256.0) -> (x-y*floor(x/y)=w408:dbl, floor(x/y)=w409:dbl)
                  n176 = Build Array(w409, w408) -> (w407:dbl[])
                  n177 = Insert Into Array(array=w405, new element=w407) -> (w406:dbl[])  [unwired: 1 in]
                }
              }
              frame 5 {
                n178 = Unbundle By Name(w415) -> ("项目信息"=w425:refnum<vi>)
                n179 = property class="Tbl (严格)"(reference=w425) -> ("Value"=w424:string[][])  [unwired: 1 in, 2 out]
                n180 = Index Array(array=w424, index (col)=1 ("禁用的索引 (列)")) -> (element=w426:string[])  [unwired: 1 in]
                n181 = Increment(x=w416) -> (x+1=w423:dbl)
                n182 = Multiply(x=w416, y=3.0) -> (x*y=w420:dbl)
                n183 = Add(x=w420, y=23.0) -> (x+y=w422:dbl)
                n184 = Array Subset(array=w426, index=w422, length=w423) -> (w428:string[])
                n185 = Fract/Exp String To Number(string=w428) -> (number=w418:dbl[])  [unwired: 4 out]
                n186 = for {
                  tunnel: w418 -> [w436] mode=indexing
                  shift-right: [w431] -> w414
                  shift-left: dbl[] [] -> [w430]
                  n187 = Quotient & Remainder(x=w436, y=256.0) -> (x-y*floor(x/y)=w433:dbl, floor(x/y)=w434:dbl)
                  n188 = Build Array(w434, w433) -> (w432:dbl[])
                  n189 = Insert Into Array(array=w430, new element=w432) -> (w431:dbl[])  [unwired: 1 in]
                }
              }
              frame 12 {
                w442 = 16 ("长度")
                # "产品编号"
                n190 = Unbundle By Name(w441) -> ("一级故障 4"=w440:refnum<vi>)
                n191 = property class="Clust (严格)"(reference=w440) -> ("Value"=w439:T3)  [unwired: 1 in, 2 out]
                n192 = Unbundle By Name(w439) -> ("产品编号"=w438:string)
                n193 = String To Byte Array(string=w438) -> (unsigned byte array=w444:u8[])
                n194 = Array Subset(array=w444, length=w442) -> (w443:u8[])  [unwired: 1 in]
              }
              frame 6 {
                w464 = 256.0 ("y")
                w466 = 256.0 ("y")
                # "电池额定容量,实际容量"
                n195 = Unbundle By Name(w455) -> ("一级故障 4"=w454:refnum<vi>)
                n196 = property class="Clust (严格)"(reference=w454) -> ("Value"=w453:T3)  [unwired: 1 in, 2 out]
                n197 = Unbundle By Name(w453) -> ("电池额定容量(A)"=w451:dbl, "电池实际容量(A)"=w450:dbl)
                n198 = call "输入分辨率计算-EV05.vi"("1字节?"=TRUE, "数值 2"=w450, "数值"=w451, "分辨率"=0.1) -> ("高字节 2"=w448:dbl, "高字节1"=w449:dbl)  [unwired: 1 in, 5 out]
                n199 = Quotient & Remainder(x=w449, y=w466) -> (x-y*floor(x/y)=w470:dbl, floor(x/y)=w472:dbl)
                n200 = Quotient & Remainder(x=w448, y=w464) -> (x-y*floor(x/y)=w457:dbl, floor(x/y)=w461:dbl)
                n201 = Quotient & Remainder(x=w472, y=w466) -> (x-y*floor(x/y)=w469:dbl, floor(x/y)=w471:dbl)
                n202 = Quotient & Remainder(x=w461, y=w464) -> (x-y*floor(x/y)=w458:dbl, floor(x/y)=w462:dbl)
                n203 = Quotient & Remainder(x=w471, y=w466) -> (x-y*floor(x/y)=w468:dbl, floor(x/y)=w467:dbl)
                n204 = Quotient & Remainder(x=w462, y=w464) -> (x-y*floor(x/y)=w459:dbl, floor(x/y)=w463:dbl)
                n205 = Quotient & Remainder(x=w467, y=w466) -> (x-y*floor(x/y)=w465:dbl)  [unwired: 1 out]
                n206 = Quotient & Remainder(x=w463, y=w464) -> (x-y*floor(x/y)=w460:dbl)  [unwired: 1 out]
                n207 = Build Array(w465, w468, w469, w470, w460, w459, w458, w457) -> (w474:dbl[])
              }
              frame 7 {
                # "SOC"
                n208 = Unbundle By Name(w482) -> ("一级故障 4"=w483:refnum<vi>)
                n209 = property class="Clust (严格)"(reference=w483) -> ("Value"=w481:T3)  [unwired: 1 in, 2 out]
                n210 = Unbundle By Name(w481) -> ("SOC(%)"=w479:dbl)
                n211 = call "输入分辨率计算-EV05.vi"("1字节?"=FALSE, "数值"=w479, "分辨率"=0.1) -> ("低字节"=w476:dbl, "高字节1"=w477:dbl)  [unwired: 2 in, 5 out]
                n212 = Build Array(w477, w476) -> (w486:dbl[])
              }
              frame 8 {
                w492 = 8 ("长度")
                # "配置文件版本"
                n213 = Unbundle By Name(w490) -> ("一级故障 4"=w491:refnum<vi>)
                n214 = property class="Clust (严格)"(reference=w491) -> ("Value"=w489:T3)  [unwired: 1 in, 2 out]
                n215 = Unbundle By Name(w489) -> ("配置文件版本"=w488:string)
                n216 = String To Byte Array(string=w488) -> (unsigned byte array=w494:u8[])
                n217 = Array Subset(array=w494, length=w492) -> (w493:u8[])  [unwired: 1 in]
              }
              frame 9 {
                n218 = Unbundle By Name(w500) -> ("一级故障 4"=w506:refnum<vi>)
                n219 = property class="Clust (严格)"(reference=w506) -> ("Value"=w505:T3)  [unwired: 1 in, 2 out]
                n220 = Unbundle By Name(w505) -> ("使用者"=w504:dbl)
                n221 = Quotient & Remainder(x=w504, y=256.0) -> (x-y*floor(x/y)=w501:dbl, floor(x/y)=w502:dbl)
                n222 = call "当前时间解析-8.6.vi"("需要秒？(T)"=TRUE) -> ("年"=w512:u8, "月"=w511:u8, "日"=w510:u8, "时"=w509:u8, "分"=w508:u8, "秒"=w507:u8)  [unwired: 13 out]
                n223 = Build Array(w502, w501, w512, w511, w510, w509, w508, w507) -> (w499:dbl[])
              }
              frame 10 {
                w519 = 8 ("长度")
                # "车牌号"
                n224 = Unbundle By Name(w517) -> ("一级故障 4"=w518:refnum<vi>)
                n225 = property class="Clust (严格)"(reference=w518) -> ("Value"=w516:T3)  [unwired: 1 in, 2 out]
                n226 = Unbundle By Name(w516) -> ("车架(牌)号"=w515:string)
                n227 = String To Byte Array(string=w515) -> (unsigned byte array=w521:u8[])
                n228 = Array Subset(array=w521, length=w519) -> (w520:u8[])  [unwired: 1 in]
              }
              frame 11 {
                # "SOH"
                n229 = Unbundle By Name(w530) -> ("一级故障 4"=w531:refnum<vi>)
                n230 = property class="Clust (严格)"(reference=w531) -> ("Value"=w529:T3)  [unwired: 1 in, 2 out]
                n231 = Unbundle By Name(w529) -> ("SOH(%)"=w528:dbl)
                n232 = call "输入分辨率计算-EV05.vi"("1字节?"=FALSE, "数值"=w528, "分辨率"=0.1) -> ("低字节"=w524:dbl, "高字节1"=w525:dbl)  [unwired: 2 in, 5 out]
                n233 = Build Array(w525, w524) -> (w534:dbl[])
              }
            }
          }
        }
        frame "产品编号" {
          w546 = 16 ("长度")
          # "产品编号"
          n234 = Unbundle By Name(w548) -> ("一级故障 4"=w540:refnum<vi>)
          n235 = property class="Clust (严格)"(reference=w540) -> ("Value"=w539:T3)  [unwired: 1 in, 2 out]
          n236 = Unbundle By Name(w539) -> ("产品编号"=w538:string)
          n237 = String To Byte Array(string=w538) -> (unsigned byte array=w541:u8[])
          n238 = Array Subset(array=w541, length=w546) -> (w549:u8[])  [unwired: 1 in]
          n239 = Build Array(w549) -> (w535:u8[][])
          n240 = Build Array(w546) -> (w537:i32[])
          n241 = Build Array(u32 1 ("命令序号")) -> (w536:u32[])
          n242 = Build Array("产品编号") -> (w542:string[])
        }
        frame "二维码" {
          w562 = 30 ("长度")
          # "产品编号"
          n243 = local read "主板二维码"() -> (w553:string)
          n244 = Search and Replace String(input string=w553, search string="BNET" ("搜索字符串"), replace string="") -> (result string=w550:string)  [unwired: 5 in, 3 out]
          n245 = String To Byte Array(string=w550) -> (unsigned byte array=w557:u8[])
          n246 = Array Subset(array=w557, length=w562) -> (w564:u8[])  [unwired: 1 in]
          n247 = Build Array(w564) -> (w554:u8[][])
          n248 = Build Array(w562) -> (w556:i32[])
          n249 = Build Array(u32 1 ("命令序号")) -> (w555:u32[])
          n250 = Build Array("写二维码") -> (w558:string[])
        }
        frame "电压个数" {
          w566 = 0 ("索引")
          # "电压个数"
          n251 = Unbundle By Name(w586) -> ("项目信息"=w580:refnum<vi>)
          n252 = property class="Tbl (严格)"(reference=w580) -> ("Value"=w579:string[][])  [unwired: 1 in, 2 out]
          n253 = Index Array(array=w579, index (col)=1 ("禁用的索引 (列)")) -> (element=w581:string[])  [unwired: 1 in]
          n254 = Increment(x=w567) -> ()  [unwired: 1 out]
          n255 = Array Subset(array=w581, index=0 ("索引"), length=w567) -> (w583:string[])
          n256 = Fract/Exp String To Number(string=w583) -> (number=w574:dbl[])  [unwired: 4 out]
          n257 = for {
            tunnel: w574 -> [w594] mode=indexing
            shift-right: [w589] -> w572
            shift-left: dbl[] [] -> [w588]
            n258 = Quotient & Remainder(x=w594, y=256.0) -> (x-y*floor(x/y)=w591:dbl, floor(x/y)=w592:dbl)
            n259 = Build Array(w592, w591) -> (w590:dbl[])
            n260 = Insert Into Array(array=w588, new element=w590) -> (w589:dbl[])  [unwired: 1 in]
          }
          n261 = Build Array(63.0 ("元素")) -> (w578:dbl[])
          n262 = Insert Into Array(array=w572, index=w566, new element #1=w567, new element #2=w566, new element #3=1.0 ("新元素/子数组")) -> (w587:dbl[])
          n263 = Build Array(u32 2 ("命令序号")) -> (w576:u32[])
          n264 = Build Array(w587) -> (w571:dbl[][])
          n265 = Build Array("电压个数") -> (w568:string[])
        }
        frame "电压起始值" {
          n266 = Unbundle By Name(w616) -> ("项目信息"=w611:refnum<vi>)
          n267 = property class="Tbl (严格)"(reference=w611) -> ("Value"=w610:string[][])  [unwired: 1 in, 2 out]
          n268 = Index Array(array=w610, index (col)=1 ("禁用的索引 (列)")) -> (element=w612:string[])  [unwired: 1 in]
          n269 = Add(x=21.0, y=w599) -> (x+y=w601:dbl)
          n270 = Increment(x=w599) -> (x+1=w598:dbl)
          n271 = Array Subset(array=w612, index=w601, length=w598) -> (w614:string[])
          n272 = Fract/Exp String To Number(string=w614) -> (number=w604:dbl[])  [unwired: 4 out]
          n273 = for {
            tunnel: w604 -> [w623] mode=indexing
            shift-right: [w618] -> w602
            shift-left: dbl[] [] -> [w617]
            n274 = Quotient & Remainder(x=w623, y=256.0) -> (x-y*floor(x/y)=w620:dbl, floor(x/y)=w621:dbl)
            n275 = Build Array(w621, w620) -> (w619:dbl[])
            n276 = Insert Into Array(array=w617, new element=w619) -> (w618:dbl[])  [unwired: 1 in]
          }
          n277 = Build Array(62.0 ("元素")) -> (w608:dbl[])
          n278 = Build Array(u32 4 ("命令序号")) -> (w606:u32[])
          n279 = Build Array(w602) -> (w609:dbl[][])
          n280 = Build Array("电压起始值") -> (w595:string[])
        }
        frame "通道电压数" {
          n281 = Unbundle By Name(w643) -> ("项目信息"=w638:refnum<vi>)
          n282 = property class="Tbl (严格)"(reference=w638) -> ("Value"=w637:string[][])  [unwired: 1 in, 2 out]
          n283 = Index Array(array=w637, index (col)=1 ("禁用的索引 (列)")) -> (element=w639:string[])  [unwired: 1 in]
          n284 = Increment(x=w630) -> (x+1=w629:dbl)
          n285 = Array Subset(array=w639, index=w629, length=20 ("长度")) -> (w641:string[])
          n286 = Fract/Exp String To Number(string=w641) -> (number=w625:dbl[])  [unwired: 4 out]
          n287 = for {
            tunnel: w625 -> [w645] mode=indexing
            tunnel: [w644] -> w624 mode=indexing
            w646 = 12.0 ("y")
            n288 = Greater?(x=w645, y=w646) -> (0:w647:bool)
            n289 = Select(t=w646, s=w647, f=w645) -> (s? t:f=w644:dbl)
          }
          n290 = Build Array(w624) -> (w636:dbl[][])
          n291 = Build Array(20.0 ("元素")) -> (w635:dbl[])
          n292 = Build Array(u32 3 ("命令序号")) -> (w633:u32[])
          n293 = Build Array("通道电压数") -> (w626:string[])
        }
        frame "温度个数" {
          w648 = 0 ("索引")
          n294 = Unbundle By Name(w671) -> ("项目信息"=w666:refnum<vi>)
          n295 = property class="Tbl (严格)"(reference=w666) -> ("Value"=w665:string[][])  [unwired: 1 in, 2 out]
          n296 = Index Array(array=w665, index (col)=1 ("禁用的索引 (列)")) -> (element=w667:string[])  [unwired: 1 in]
          n297 = Multiply(x=w651, y=2.0) -> (x*y=w652:dbl)
          n298 = Add(x=w652, y=22.0) -> ()  [unwired: 1 out]
          n299 = Array Subset(array=w667, index=w651, length=w651) -> (w669:string[])
          n300 = Fract/Exp String To Number(string=w669) -> (number=w658:dbl[])  [unwired: 4 out]
          n301 = for {
            tunnel: w658 -> [w678] mode=indexing
            shift-right: [w673] -> w650
            shift-left: dbl[] [] -> [w672]
            n302 = Quotient & Remainder(x=w678, y=256.0) -> (x-y*floor(x/y)=w675:dbl, floor(x/y)=w676:dbl)
            n303 = Build Array(w676, w675) -> (w674:dbl[])
